vi "write TBM configuration.vi"(8 "error in":errorcluster, 10 "configuration":refnum<class "TBM configuration.lvclass">, 11 "Watchdog editor node in":refnum<class "Watchdog editor node.lvclass">) -> (0 "error out":errorcluster, 3 "Watchdog editor node out":refnum<class "Watchdog editor node.lvclass">)   [LabVIEW 2013, in "Watchdog editor node.lvclass"]
uses:
  Watchdog editor node.lvclass
  <vilib>/NI/Tag Bus Module Framework/root configuration/TBM configuration.lvclass
  module/configuration/Watchdog configuration.lvclass
  Watchdog editor node.lvclass/Watchdog editor node.ctl
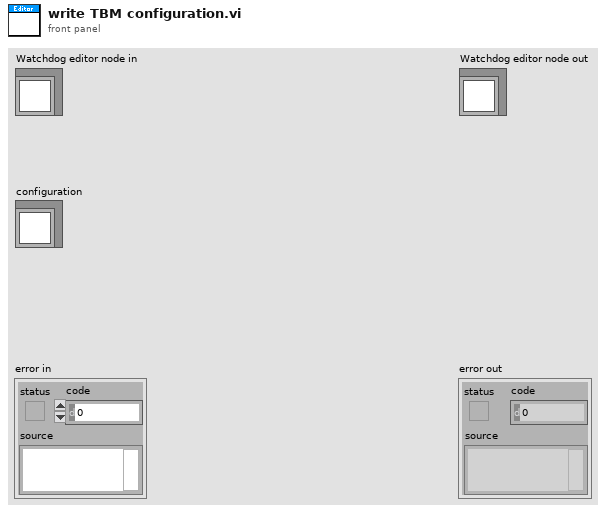
[diagram p1: front panel]
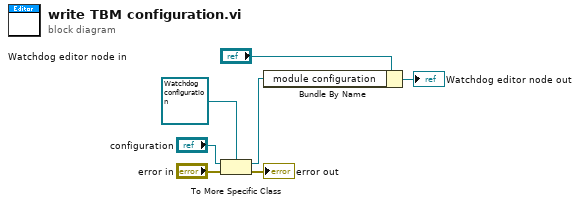
[diagram p0: block diagram]
diagram:
  n1 = To More Specific Class(target class=refnum<class "Watchdog configuration.lvclass"> refnum ("module configuration"), reference="configuration", error in="error in") -> (specific class reference=w1:refnum<class "Watchdog configuration.lvclass">, error out=→"error out":errorcluster)
  n2 = Bundle By Name(cluster="Watchdog editor node in", "module configuration"=w1) -> (→"Watchdog editor node out":refnum<class "Watchdog editor node.lvclass">)
